vi "Configure Trigger (Transition).vi"(0 "VISA resource name":refnum<visa-resource-name>, 1 "Low Threshold (0.001 V)":dbl=0.001, 2 "High Threshold (0.01 V)":dbl=0.01, 5 "Trigger Source (1: Channel 1)":i32(ring)=1 items=["Channel 1"=1, "Channel 2"=2, "Channel 3"=3, "Channel 4"=4], 7 "Trigger Polarity (0: Rising)":i32(ring) items=["Rising", "Falling"], 9 "Violation Mode (0: Greater Than)":i32(ring) items=["Greater Than", "Less Than"], 11 "error in (no error)":errorcluster, 12 "Time Limit (1.5E-9)":dbl=1.5e-09) -> (4 "VISA resource name out":refnum<visa-resource-name>, 15 "error out":errorcluster)   [LabVIEW 2012, in "Agilent 8000 Series.lvlib"]
doc: "Configures the transition violation trigger. It configures the trigger source, and the transition violation properties."
uses:
  Agilent 8000 Series.lvlib
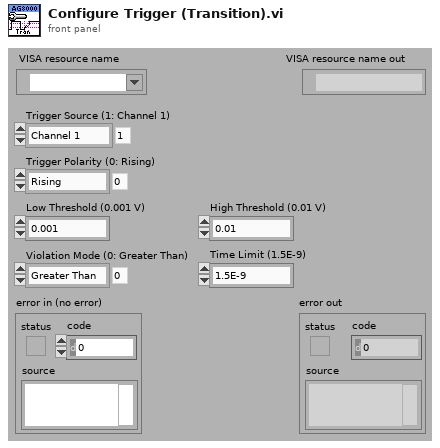
[diagram p1: front panel]
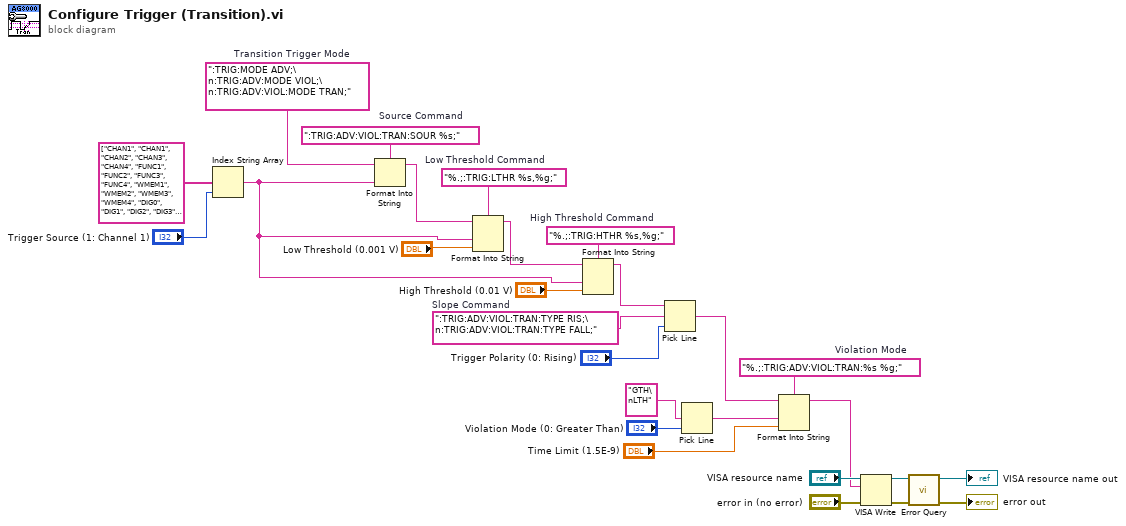
[diagram p0: block diagram]
diagram:
  w5 = "%.;:TRIG:ADV:VIOL:TRAN:%s %g;"  # Violation Mode
  w12 = ":TRIG:ADV:VIOL:TRAN:TYPE RIS;\n:TRIG:ADV:VIOL:TRAN:TYPE FALL;"  # Slope Command
  w15 = "%.;:TRIG:HTHR %s,%g;"  # High Threshold Command
  w16 = "%.;:TRIG:LTHR %s,%g;"  # Low Threshold Command
  w18 = ":TRIG:ADV:VIOL:TRAN:SOUR %s;"  # Source Command
  w21 = ":TRIG:MODE ADV;\n:TRIG:ADV:MODE VIOL;\n:TRIG:ADV:VIOL:MODE TRAN;"  # Transition Trigger Mode
  n1 = Index String Array(1:"Trigger Source (1: Channel 1)", 2:string[] ["CHAN1", "CHAN1", "CHAN2", "CHAN3", "CHAN4", "FUNC1", "FUNC2", "FUNC3", "FUNC4", "WMEM1", "WMEM2", "WMEM3", "WMEM4", "DIG0", "DIG1", "DIG2", "DIG3", "DIG4", "DIG5", "DIG6", "DIG7", "DIG8", "DIG9", "DIG10", "DIG11", "DIG12", "DIG13", "DIG14", "DIG15", "AUX", "LINE"]) -> (0:w1:string)  [unwired: 1 in]
  n2 = Format Into String(format string=w18, initial string=w21, w1) -> (resulting string=w17:string)  [unwired: 1 in, 1 out]
  n3 = Format Into String(format string=w16, initial string=w17, w1, "Low Threshold (0.001 V)") -> (resulting string=w14:string)  [unwired: 1 in, 1 out]
  n4 = Format Into String(format string=w15, initial string=w14, w1, "High Threshold (0.01 V)") -> (resulting string=w13:string)  [unwired: 1 in, 1 out]
  n5 = Pick Line(string ("")=w13, multi-line string=w12, line index="Trigger Polarity (0: Rising)") -> (output string=w6:string)
  n6 = Pick Line(multi-line string="GTH\nLTH" ("Command"), line index="Violation Mode (0: Greater Than)") -> (output string=w7:string)  [unwired: 1 in]
  n7 = Format Into String(format string=w5, initial string=w6, w7, "Time Limit (1.5E-9)") -> (resulting string=w4:string)  [unwired: 1 in, 1 out]
  n8 = VISA Write(VISA resource name="VISA resource name", write buffer=w4, error in (no error)="error in (no error)") -> (VISA resource name out=w23:refnum<visa-resource-name>, error out=w22:errorcluster)  [unwired: 1 out]
  n9 = call "Error Query.vi"("error in (no error)"=w22, "VISA resource name"=w23) -> ("error out"=→"error out":errorcluster, "VISA resource name out"=→"VISA resource name out":refnum<visa-resource-name>)  [unwired: 6 in, 2 out]
